vi "lab4_copy.vi"() -> ()   [LabVIEW 2017]
panel:
  out "2D Picture":picture
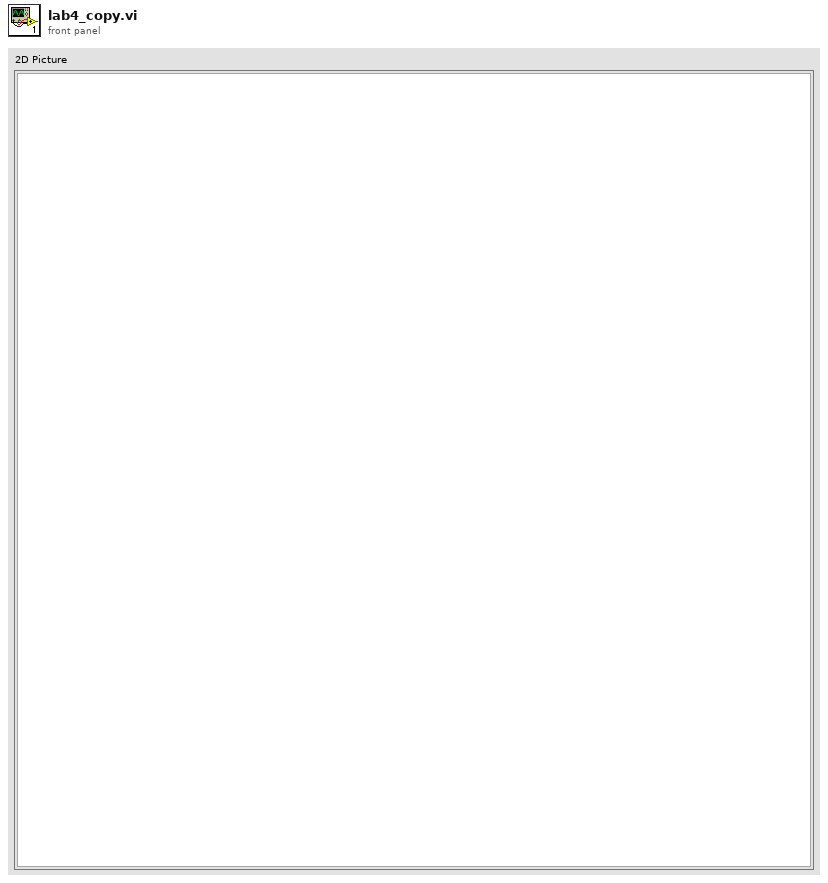
[diagram p1: front panel]
types:
  T1 = cluster{"Width":u16, "Style":enum32{"Solid", "Dash", "Dot", "DashDot", "DashDotDot"}}
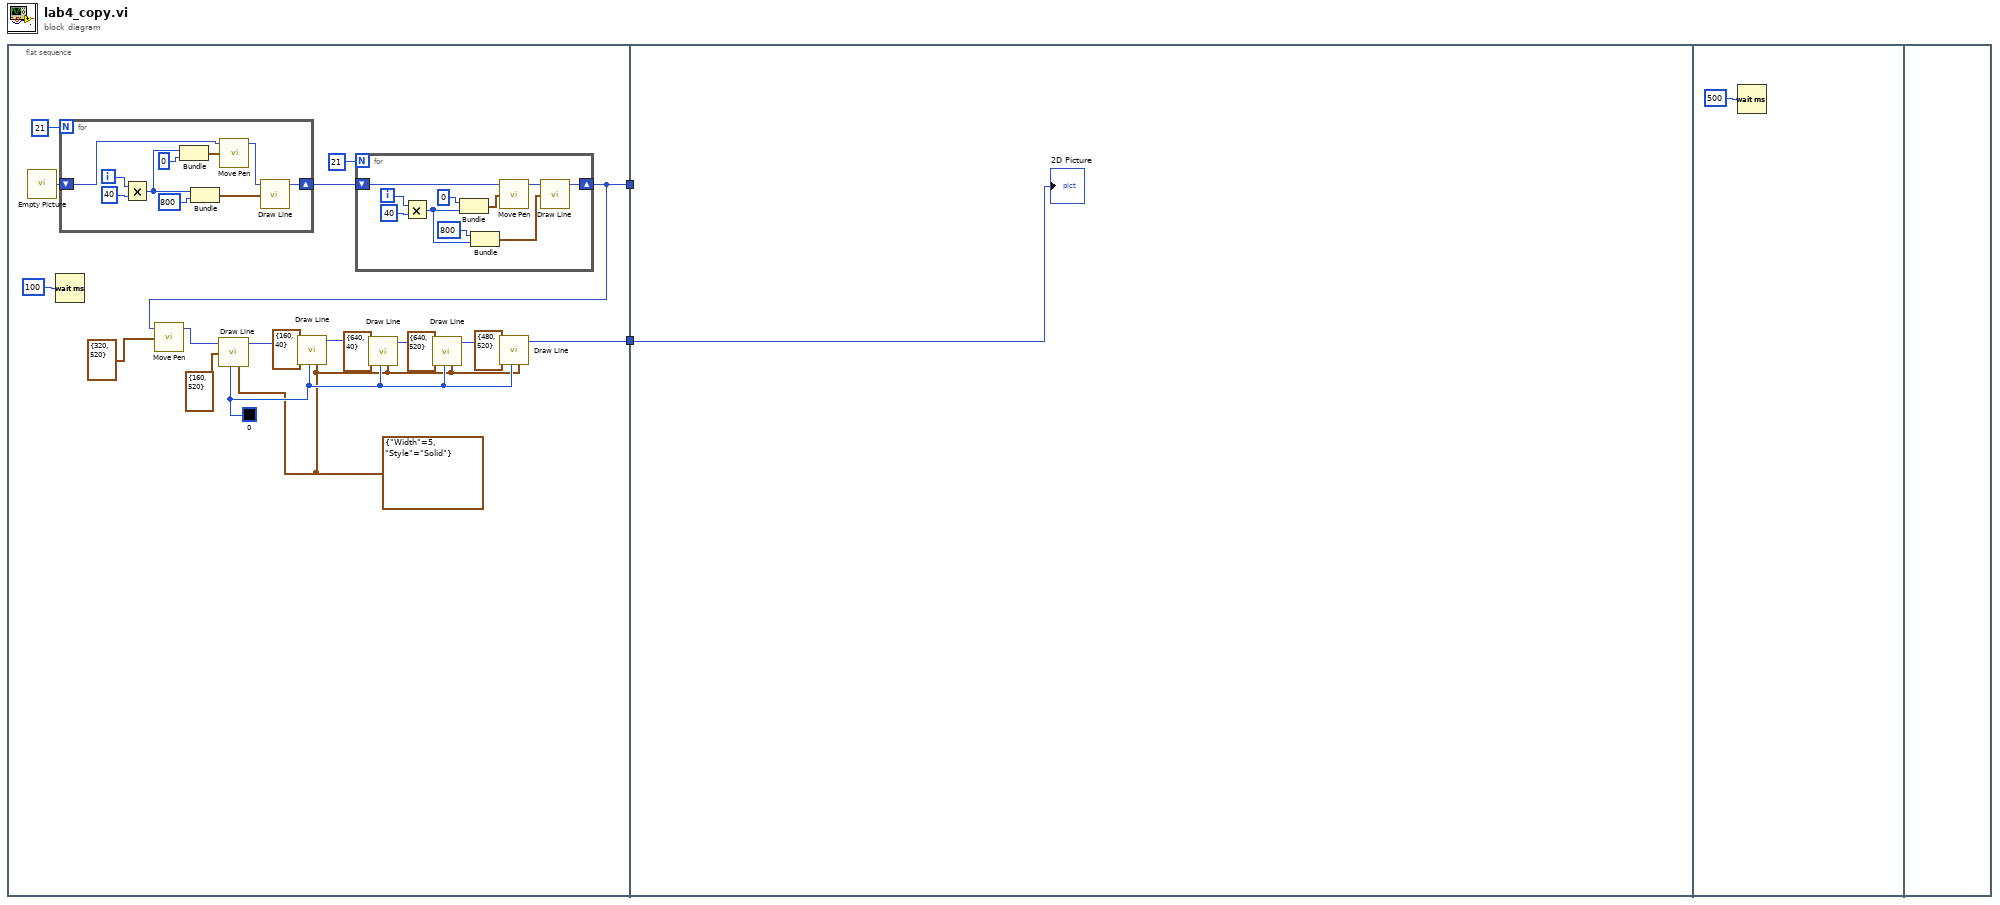
[diagram p0: block diagram]
diagram:
  n1 = flat-sequence {
    tunnel: [w8] -> w2
    tunnel: [w3] -> w1
    tunnel: w2 -> [_]
    tunnel: w1 -> [w43]
    frame #0 {
      w10 = u32 0 ("color(black)")
      w9 = T1 {"Width"=5, "Style"=enum."Solid"} ("pen")
      n2 = call "Empty Picture"() -> ("empty picture"=w20:picture)
      n3 = Wait (ms)(milliseconds to wait=u32 100) -> ()  [unwired: 1 out]
      n4 = for {
        N: 21 -> [_]
        shift-right: [w40] -> w18
        shift-left: w20 -> [w41]
        i -> [w33]
        n5 = Multiply(x=w33, y=i16 40 ("x 2")) -> (x*y=w34:i32)
        n6 = Bundle(w34, 0) -> (w37:cluster{i32, i32})  [unwired: 1 in]
        n7 = Bundle(w34, 800) -> (w35:cluster{i32, i32})  [unwired: 1 in]
        n8 = call <vilib>:"Move Pen.vi"("new position"=w37, "picture"=w41) -> ("new picture"=w42:picture)  [unwired: 3 in]
        n9 = call <vilib>:"Draw Line.vi"("picture"=w42, "end point"=w35) -> ("new picture"=w40:picture)  [unwired: 7 in]
      }
      n10 = for {
        N: 21 -> [_]
        shift-right: [w30] -> w8
        shift-left: w18 -> [w31]
        i -> [w26]
        n11 = Multiply(x=w26, y=i16 40 ("x 2")) -> (x*y=w23:i32)
        n12 = Bundle(0, w23) -> (w28:cluster{i32, i32})  [unwired: 1 in]
        n13 = Bundle(800, w23) -> (w27:cluster{i32, i32})  [unwired: 1 in]
        n14 = call <vilib>:"Move Pen.vi"("new position"=w28, "picture"=w31) -> ("new picture"=w32:picture)  [unwired: 3 in]
        n15 = call <vilib>:"Draw Line.vi"("picture"=w32, "end point"=w27) -> ("new picture"=w30:picture)  [unwired: 7 in]
      }
      n16 = call <vilib>:"Move Pen.vi"("new position"=cluster{"x":i16, "y":i16} {"x"=320, "y"=520}, "picture"=w8) -> ("new picture"=w16:picture)  [unwired: 3 in]
      n17 = call <vilib>:"Draw Line.vi"("picture"=w16, "end point"=cluster{"x":i16, "y":i16} {"x"=160, "y"=520}, "color(black)"=w10, "pen"=w9) -> ("new picture"=w14:picture)  [unwired: 5 in]
      n18 = call <vilib>:"Draw Line.vi"("picture"=w14, "end point"=cluster{"x":i16, "y":i16} {"x"=160, "y"=40}, "color(black)"=w10, "pen"=w9) -> ("new picture"=w13:picture)  [unwired: 5 in]
      n19 = call <vilib>:"Draw Line.vi"("picture"=w13, "end point"=cluster{"x":i16, "y":i16} {"x"=640, "y"=40}, "color(black)"=w10, "pen"=w9) -> ("new picture"=w12:picture)  [unwired: 5 in]
      n20 = call <vilib>:"Draw Line.vi"("picture"=w12, "end point"=cluster{"x":i16, "y":i16} {"x"=640, "y"=520}, "color(black)"=w10, "pen"=w9) -> ("new picture"=w11:picture)  [unwired: 5 in]
      n21 = call <vilib>:"Draw Line.vi"("picture"=w11, "end point"=cluster{"x":i16, "y":i16} {"x"=480, "y"=520}, "color(black)"=w10, "pen"=w9) -> ("new picture"=w3:picture)  [unwired: 5 in]
    }
    frame #1 {
      "2D Picture" <- w43
    }
    frame #2 {
      n22 = Wait (ms)(milliseconds to wait=u32 500) -> ()  [unwired: 1 out]
    }
    frame #3 {
    }
  }
